vi "Test_WriteValue_InvalidType_Error.vi"(8 "error in (no error)":errorcluster, 11 "TestCase in":refnum<class "TestStreamToDiskTransport.lvclass">) -> (0 "error out":errorcluster, 3 "TestCase out":refnum<class "TestStreamToDiskTransport.lvclass">)   [LabVIEW 2017, in "TestStreamToDiskTransport.lvclass"]
uses:
  TestStreamToDiskTransport.lvclass
  TestStreamToDiskTransport.lvclass/TestStreamToDiskTransport.ctl
  Source/Concrete/StreamToDiskTransport/StreamToDiskTransport.lvclass/StreamToDiskTransport.ctl
  <vilib>/Utility/error.llb/Clear Errors.vi
  Source/Concrete/StreamToDiskTransport/StreamToDiskTransport.lvclass
  C:/Git/composed-transport/Source/ITransport/ITransport.lvclass
  Source/ITransport/ITransport.lvclass
panel:
  out "Return Error":errorcluster
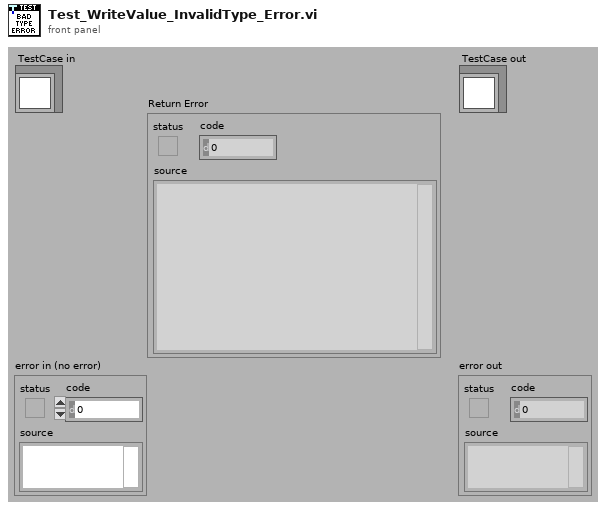
[diagram p1: front panel]
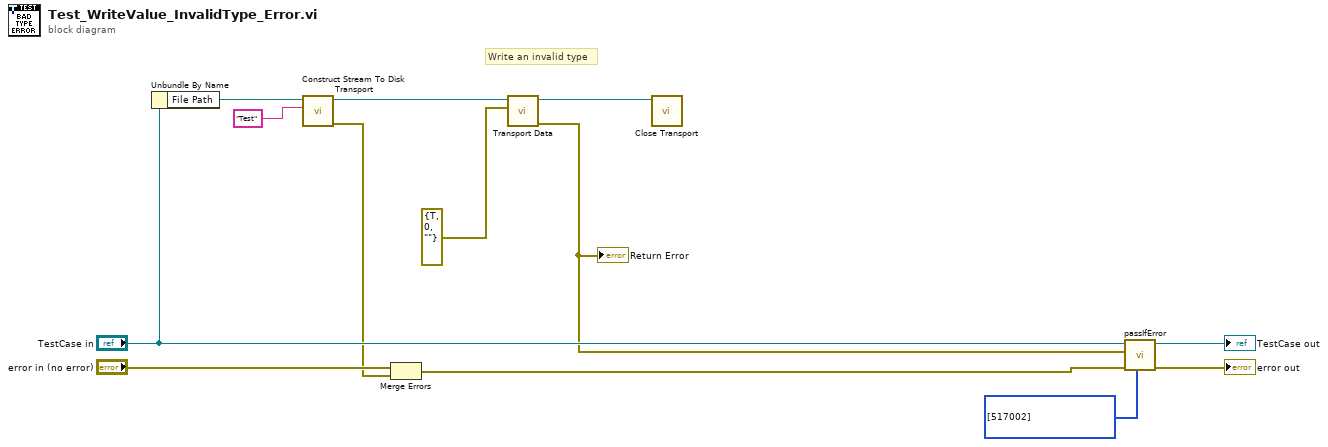
[diagram p0: block diagram]
diagram:
  # "Write an invalid type"
  n1 = Unbundle By Name("TestCase in") -> ("File Path"=w6:path)
  n2 = call "Construct Stream To Disk Transport.vi"("Channel Name"="Test" ("Section Name"), "File Path"=w6) -> ("error out"=w1:errorcluster, "StreamToDiskTransport"=w8:refnum<class "StreamToDiskTransport.lvclass">)  [unwired: 8 in]
  n3 = Merge Errors("error in (no error)", w1) -> (w9:errorcluster)
  n4 = call "Transport Data.vi"("Value"=errorcluster {"status"=TRUE, "code"=0, "source"=""} ("Test Value"), "ITransport in"=w8) -> ("error out"=w3:errorcluster, "ITransport out"=w13:refnum<class "StreamToDiskTransport.lvclass">)  [unwired: 8 in]
  "Return Error" <- w3
  n5 = call-dynamic "Close Transport.vi"("StreamToDiskTransport"=w13) -> ()  [unwired: 10 in, 1 out]
  n6 = call-dynamic "passIfError.vi"("passing error codes (default = any error code)"=i32[] [517002], "error in (no error)"=w9, "error"=w3, "TestCase in"="TestCase in") -> ("error out"=→"error out":errorcluster, "TestCase out"=→"TestCase out":refnum<class "TestStreamToDiskTransport.lvclass">)  [unwired: 6 in]
